vi "Cmd.ReadResp.vi"(7 "IgnoreError":bool, 8 "error in (no error)":errorcluster, 9 "Timeout [ms] (1000)":i32=1000, 10 "Request":string, 11 "connection ID":refnum<k5>) -> (0 "error out":errorcluster, 2 "ResponseParameters":string, 3 "connection ID out":refnum<k5>)   [LabVIEW 2016]
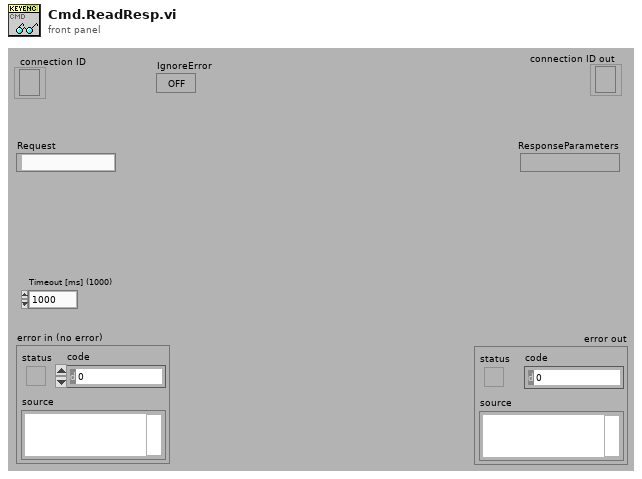
[diagram p1: front panel]
types:
  T1 = enum16{"Standard", "Buffered", "CRLF", "Immediate"}
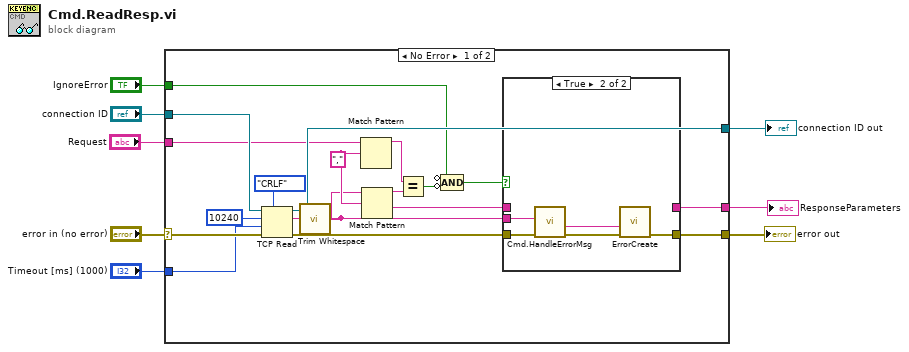
[diagram p0: block diagram]
diagram:
  n1 = case shown="No Error" "error in (no error)" {
    selector: "error in (no error)" -> [w26 w35]
    tunnel: [w22 w35] -> w8
    tunnel: "Timeout [ms] (1000)" -> [w25 _]
    tunnel: "connection ID" -> [w27 w34]
    tunnel: [w24 w34] -> w5
    tunnel: "Request" -> [w21 _]
    tunnel: [w12 _] -> w2
    tunnel: "IgnoreError" -> [w11 _]
    frame No Error {
      w20 = ","
      n2 = TCP Read(connection ID=w27, bytes to read=10240, error in (no error)=w26, 7:T1."CRLF" ("mode (standard)"), 9:w25) -> (connection ID out=w24:refnum<k5>, data out=w14:string, error out=w23:errorcluster)
      n3 = call <vilib>:"Trim Whitespace.vi"("string"=w14) -> ("trimmed string"=w13:string)  [unwired: 1 in]
      n4 = Match Pattern(string=w21, regular expression=w20) -> (before substring=w19:string)  [unwired: 1 in, 3 out]
      n5 = Match Pattern(string=w13, regular expression=w20) -> (before substring=w18:string, after substring=w17:string)  [unwired: 1 in, 2 out]
      n6 = Equal?(x=w19, y=w18) -> (x = y?=w10:bool)
      n7 = Compound Arithmetic op=AND(invert w11, invert w10) -> (w9:bool)
      n8 = case shown="True" w9 {
        tunnel: w23 -> [w29 w33]
        tunnel: [w29 w32] -> w22
        tunnel: w13 -> [_ w31]
        tunnel: w17 -> [w28 _]
        tunnel: [w28 _] -> w12
        frame False {
        }
        frame True {
          n9 = call "Cmd.HandleErrorMsg.vi"("Response"=w31) -> ("ErrorMsg"=w30:string)  [unwired: 9 in]
          n10 = call "ErrorCreate.vi"("error in (no error)"=w33, "ErrorMessage"=w30) -> ("error out"=w32:errorcluster)  [unwired: 9 in]
        }
      }
    }
    frame Error {
    }
  }
  "error out" <- w8
  "connection ID out" <- w5
  "ResponseParameters" <- w2
